vi "read_frame.vi"(6 "max payload bytes (5012)":i32=5012, 9 "timeout ms (500)":i32=500, 10 "receive queue":refnum<queue>, 11 "TCP Network Connection in":refnum<k5>) -> (0 "error out":errorcluster, 1 "hangup status code (ignore)":T1 items=["ignore"=0, "normal"=1000, "going away"=1001, "protocol error"=1002, "invalid data"=1003])   [LabVIEW 2019, in "WebSocket Server Toolkit.lvlib"]
uses:
  WebSocket Server Toolkit.lvlib
  types/frame_data.ctl
  types/status_code.ctl
  types/opcode.ctl
  <vilib>/Utility/error.llb/Error Cluster From Error Code.vi
  <vilib>/ErrorRing/Error Ring.xnode
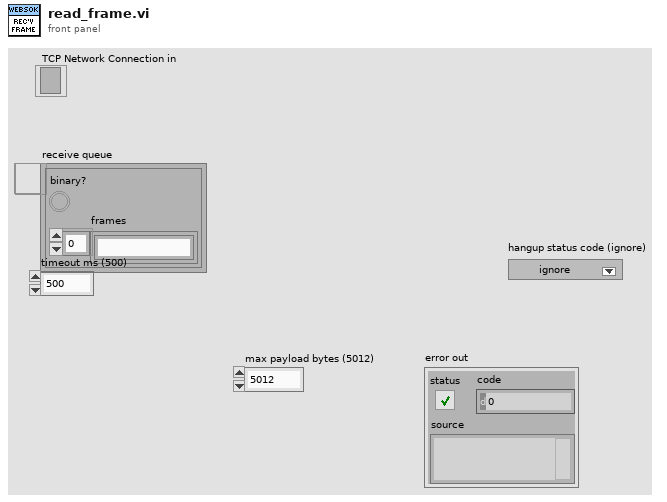
[diagram p1: front panel]
types:
  T1 = typedef "WebSocket Server Toolkit.lvlib/status_code.ctl" = u16
  T2 = typedef "WebSocket Server Toolkit.lvlib/opcode.ctl" = u8
  T3 = typedef "WebSocket Server Toolkit.lvlib/frame_data.ctl" = cluster{"binary?":bool, "frames":string[]}
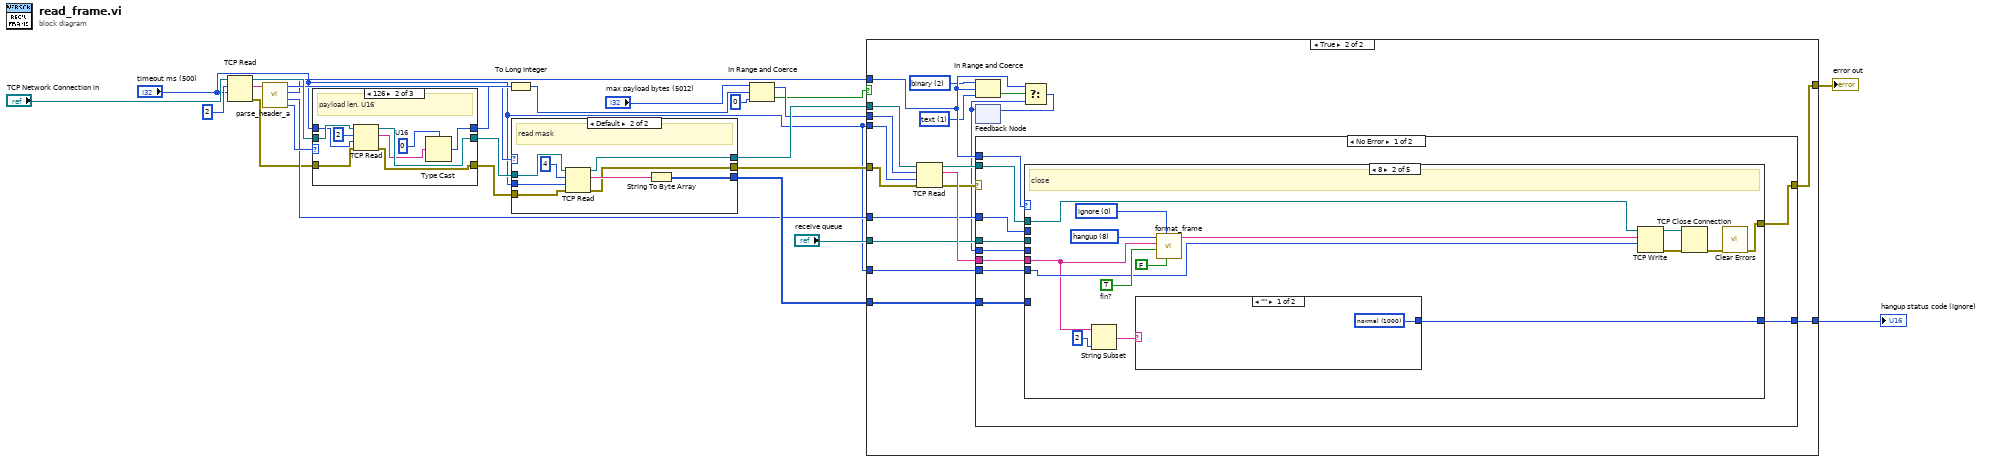
[diagram p0: block diagram]
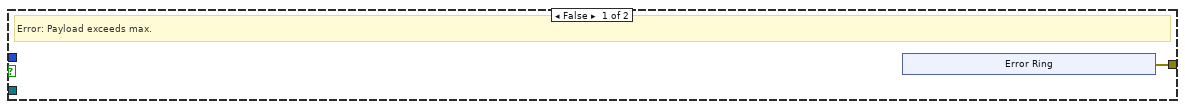
[diagram p2: hidden frame]
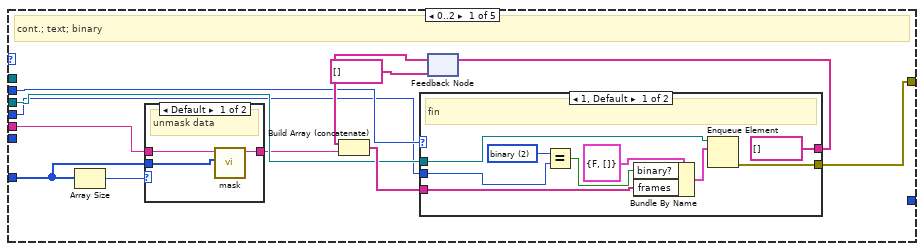
[diagram p3: hidden frame]
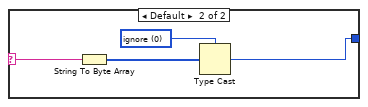
[diagram p6: hidden frame]
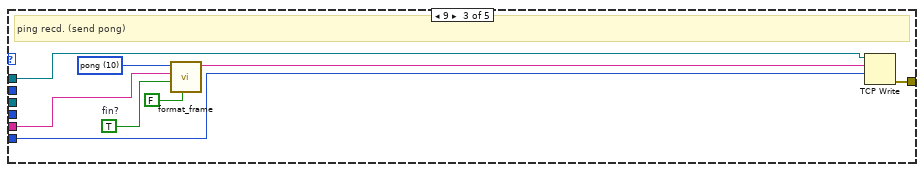
[diagram p7: hidden frame]
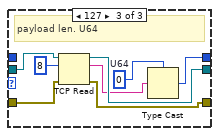
[diagram p13: hidden frame]
diagram:
  n1 = TCP Read(connection ID="TCP Network Connection in", bytes to read=2, 9:"timeout ms (500)") -> (connection ID out=w19:refnum<k5>, data out=w1:string, error out=w2:errorcluster)  [unwired: 2 in]
  n2 = call "parse_header_a.vi"("data in"=w1) -> ("payload len code"=w7:u8, "fin?"=w5:u8, "opcode"=w6:T2, "mask?"=w8:u8)  [unwired: 7 in]
  n3 = case shown="126" w7 {
    selector: w7 -> [w26 _ _]
    tunnel: w19 -> [w27 w36 w44]
    tunnel: [w27 w35 w43] -> w18
    tunnel: [w26 w31 w39] -> w14
    tunnel: w2 -> [w25 w30 w38]
    tunnel: [w25 w29 w37] -> w17
    tunnel: "timeout ms (500)" -> [_ w28 _]
    frame Default {
      # "payload len. <= 125"
    }
    frame 126 {
      w32 = u16 0  # U16
      # "payload len. U16"
      n4 = TCP Read(connection ID=w36, bytes to read=2, error in (no error)=w30, 9:w28) -> (connection ID out=w35:refnum<k5>, data out=w33:string, error out=w29:errorcluster)  [unwired: 1 in]
      n5 = Type Cast(type=w32, x=w33) -> (*(type *) &x=w31:u16)
    }
    frame 127 {
      w40 = u64 0  # U64
      # "payload len. U64"
      n6 = TCP Read(connection ID=w44, bytes to read=8, error in (no error)=w38) -> (connection ID out=w43:refnum<k5>, data out=w41:string, error out=w37:errorcluster)  [unwired: 2 in]
      n7 = Type Cast(type=w40, x=w41) -> (*(type *) &x=w39:u64)
    }
  }
  n8 = To Long Integer(number=w14) -> (32bit integer=w12:i32)
  n9 = case shown="Default" w8 {
    tunnel: w18 -> [w46 w54]
    tunnel: [w46 w53] -> w16
    tunnel: w17 -> [w45 w51]
    tunnel: [_ w49] -> w9
    tunnel: [w45 w48] -> w15
    tunnel: "timeout ms (500)" -> [_ w47]
    frame 0 {
    }
    frame Default {
      # "read mask"
      n10 = TCP Read(connection ID=w54, bytes to read=4, error in (no error)=w51, 9:w47) -> (connection ID out=w53:refnum<k5>, data out=w50:string, error out=w48:errorcluster)  [unwired: 1 in]
      n11 = String To Byte Array(string=w50) -> (unsigned byte array=w49:u8[])
    }
  }
  n12 = In Range and Coerce(upper limit="max payload bytes (5012)", x=w12, lower limit=0) -> (coerced(x)=w11:i32, In Range?=w10:bool)
  n13 = case shown="True" w10 {
    tunnel: w16 -> [_ w78]
    tunnel: w15 -> [_ w77]
    tunnel: w11 -> [_ w76]
    tunnel: [w55 w71] -> w21
    tunnel: w6 -> [_ w64]
    tunnel: w5 -> [_ w74]
    tunnel: "receive queue" -> [_ w73]
    tunnel: w9 -> [_ w70]
    tunnel: "timeout ms (500)" -> [_ w69]
    tunnel: [_ w68] -> w4
    tunnel: "timeout ms (500)" -> [_ w66]
    frame False {
      # "Error: Payload exceeds max."
      n14 = xnode "Error Ring"() -> ("error out"=w55:errorcluster)
    }
    frame True {
      w62 = T2 2 items=["continue"=0, "text"=1, "binary"=2, "hangup"=8, "ping"=9, "pong"=10] ("upper limit")
      w63 = T2 1 items=["continue"=0, "text"=1, "binary"=2, "hangup"=8, "ping"=9, "pong"=10] ("lower limit")
      n15 = TCP Read(connection ID=w78, bytes to read=w76, error in (no error)=w77, 9:w69) -> (connection ID out=w67:refnum<k5>, data out=w75:string, error out=w72:errorcluster)  [unwired: 1 in]
      n16 = In Range and Coerce(upper limit=w62, x=w64, lower limit=w63) -> (In Range?=w61:bool)  [unwired: 1 out]
      n17 = feedback #1() -> (w60:T2)  [unwired: 1 in]
      n18 = case shown="No Error" w72 {
        selector: w72 -> [_ w143]
        tunnel: w64 -> [w88 _]
        tunnel: w75 -> [w87 _]
        tunnel: w74 -> [w86 _]
        tunnel: w73 -> [w85 _]
        tunnel: [w84 w143] -> w71
        tunnel: w70 -> [w83 _]
        tunnel: [w82 _] -> w68
        tunnel: w67 -> [w81 _]
        tunnel: w66 -> [w80 _]
        tunnel: w60 -> [w79 _]
        frame No Error {
          n19 = case shown="8" w88 {
            tunnel: w87 -> [w98 w123 w139 _ _]
            tunnel: w86 -> [w97 _ _ _ _]
            tunnel: w85 -> [w94 _ _ _ _]
            tunnel: [w93 w118 w135 _ _] -> w84
            tunnel: w83 -> [w92 _ _ _ _]
            tunnel: [_ w117 _ _ _] -> w82
            tunnel: w81 -> [_ w126 w138 _ _]
            tunnel: w80 -> [_ w124 w136 _ _]
            tunnel: w79 -> [w91 _ _ _ _]
            frame 0..2 {
              # "cont.; text; binary"
              n20 = Array Size(array=w92) -> (size(s)=w90:i32)
              n21 = case shown="Default" w90 {
                tunnel: [w102 w104] -> w89
                tunnel: w98 -> [w103 w104]
                tunnel: w92 -> [w101 _]
                frame Default {
                  # "unmask data"
                  n22 = call "mask.vi"("mask"=w101, "data in"=w103) -> ("masked data"=w102:string)  [unwired: 9 in]
                }
                frame 0 {
                  # "no mask"
                }
              }
              n23 = feedback #2(string[] []) -> (w100:string[])
              n24 = Build Array (concatenate)(w100, w89) -> (w95:string[])
              n25 = case shown="1, Default" w97 {
                tunnel: [string[] [] w114] -> w96
                tunnel: w95 -> [w108 w114]
                tunnel: w94 -> [w112 _]
                tunnel: [w111 _] -> w93
                tunnel: w91 -> [w107 _]
                frame 1, Default {
                  w106 = T2 2 items=["continue"=0, "text"=1, "binary"=2, "hangup"=8, "ping"=9, "pong"=10] ("x")
                  # "fin"
                  n26 = Equal?(x=w106, y=w107) -> (x = y?=w105:bool)
                  n27 = Bundle By Name(cluster=T3 {"binary?"=FALSE, "frames"=[]} ("frame data"), "binary?"=w105, "frames"=w108) -> (w109:T3)
                  n28 = Enqueue Element(queue=w112, element=w109) -> (error out=w111:errorcluster)  [unwired: 2 in, 2 out]
                }
                frame 0 {
                  # "not fin"
                }
              }
              n29 = feedback-in #2(w96) -> ()
            }
            frame 8 {
              w116 = T1 0 items=["ignore"=0, "normal"=1000, "going away"=1001, "protocol error"=1002, "invalid data"=1003] ("hangup status code")
              w129 = TRUE  # fin?
              w128 = T2 8 items=["continue"=0, "text"=1, "binary"=2, "hangup"=8, "ping"=9, "pong"=10] ("opcode")
              # "close"
              n30 = String Subset(string=w123, length (rest)=2 ("length (rest)")) -> (substring=w115:string)  [unwired: 1 in]
              n31 = case shown="\"\"" w115 {
                selector: w115 -> [_ w131]
                tunnel: [w130 w132] -> w117
                frame "" {
                  w130 = T1 1000 items=["ignore"=0, "normal"=1000, "going away"=1001, "protocol error"=1002, "invalid data"=1003] ("hangup status code (ignore)")
                }
                frame Default {
                  w133 = T1 0 items=["ignore"=0, "normal"=1000, "going away"=1001, "protocol error"=1002, "invalid data"=1003] ("hangup status code (ignore)")
                  n32 = String To Byte Array(string=w131) -> (unsigned byte array=w134:u8[])
                  n33 = Type Cast(type=w133, x=w134) -> (*(type *) &x=w132:T1)
                }
              }
              n34 = call "format_frame.vi"("mask?"=FALSE, "hangup status code"=w116, "fin?"=w129, "data in"=w123, "opcode"=w128) -> ("frame data out"=w125:string)  [unwired: 6 in]
              n35 = TCP Write(connection ID=w126, data in=w125, 9:w124) -> (connection ID out=w120:refnum<k5>, error out=w121:errorcluster)  [unwired: 1 in, 1 out]
              n36 = TCP Close Connection(connection ID=w120, error in (no error)=w121) -> (error out=w119:errorcluster)  [unwired: 1 in, 1 out]
              n37 = call <vilib>:"Clear Errors.vi"("error in (no error)"=w119) -> ("error out"=w118:errorcluster)  [unwired: 5 in, 1 out]
            }
            frame 9 {
              w142 = TRUE  # fin?
              w141 = T2 10 items=["continue"=0, "text"=1, "binary"=2, "hangup"=8, "ping"=9, "pong"=10] ("opcode")
              # "ping recd. (send pong)"
              n38 = call "format_frame.vi"("mask?"=FALSE, "fin?"=w142, "data in"=w139, "opcode"=w141) -> ("frame data out"=w137:string)  [unwired: 7 in]
              n39 = TCP Write(connection ID=w138, data in=w137, 9:w136) -> (error out=w135:errorcluster)  [unwired: 1 in, 2 out]
            }
            frame 10 {
              # "pong recd. (do nothing)"
            }
            frame Default {
              # "unk. opcode"
            }
          }
        }
        frame Error {
        }
      }
      n40 = Select(t=w64, s=w61, f=w60) -> (s? t:f=w65:T2)
      n41 = feedback-in #1(w65) -> ()
    }
  }
  "error out" <- w21
  "hangup status code (ignore)" <- w4
